vi "Selection.vi"(11 "Population[]":T1[](array[typedef])=[{"Distance"=319.06102146675653, "Tour"=[92, 59, 43, 30, 24, 44, 41, 59, 56, 10, 3, 10, 70]}, {"Distance"=410.80789988124224, "Tour"=[70, 59, 92, 30, 24, 44, 56, 59, 10, 10, 3, 41, 43]}, {"Distance"=451.4455043022414, "Tour"=[92, 59, 43, 30, 24, 44, 41, 59, 56, 10, 70, 10, 3]}, {"Distance"=482.02041504678834, "Tour"=[92, 59, 43, 30, 59, 44, 56, 10, 41, 24, 3, 10, 70]}, {"Distance"=488.92486714516036, "Tour"=[59, 59, 43, 30, 24, 44, 41, 92, 56, 10, 3, 10, 70]}]) -> (3 "Range":cluster{dbl, dbl}[](array[cluster]))   [LabVIEW 2015, in "TSP Library.lvlib"]
uses:
  TSP Library.lvlib
  TypeDef/Path.ctl
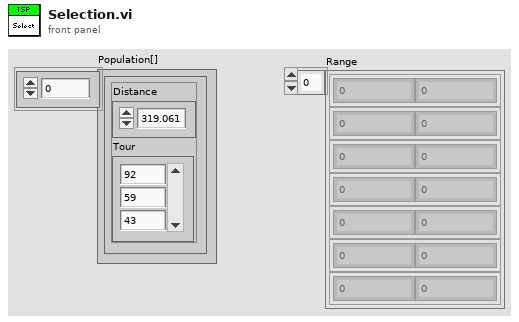
[diagram p1: front panel]
types:
  T1 = typedef "TSP Library.lvlib/Path.ctl" = cluster{"Distance":dbl, "Tour":u16[]}
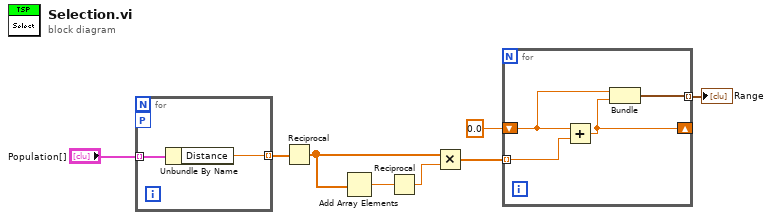
[diagram p0: block diagram]
diagram:
  n1 = for {
    tunnel: "Population[]" -> [w10] mode=indexing
    tunnel: [w9] -> w7 mode=indexing
    workers-P: _ -> [_]
    n2 = Unbundle By Name(w10) -> ("Distance"=w9:dbl)
  }
  n3 = Reciprocal(x=w7) -> (1/x=w5:dbl[])
  n4 = Add Array Elements(numeric array=w5) -> (sum=w6:dbl)
  n5 = Reciprocal(x=w6) -> (1/x=w4:dbl)
  n6 = Multiply(x=w5, y=w4) -> (x*y=w3:dbl[])
  n7 = for {
    tunnel: w3 -> [w13] mode=indexing
    shift-right: [w11] -> _
    shift-left: 0.0 -> [w14]
    tunnel: [w12] -> w1 mode=indexing
    n8 = Add(x=w14, y=w13) -> (x+y=w11:dbl)
    n9 = Bundle(w14, w11) -> (w12:cluster{dbl, dbl})  [unwired: 1 in]
  }
  "Range" <- w1
